vi "Button Toggle Motor.vi"(8 "error in (no error)":errorcluster, 9 "Motor Power":dbl format="%#_13g", 10 "refnum name":string="My Motor RefNum", 11 "Input":bool) -> (0 "error out":errorcluster)   [LabVIEW 2016, in "Huskie Swerve.lvlib"]
uses:
  Huskie Swerve.lvlib
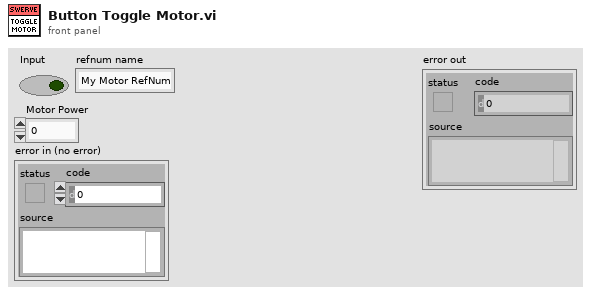
[diagram p1: front panel]
types:
  T1 = typedef "WPI_MotorControlDeviceRef.ctl" = cluster{"DeviceStatus":errorcluster, "Type":T2, "PWM":cluster{"PWM Channel":T3, "DeadBand":T4}, "CAN":cluster{"Device Number":u8, "SetOutput VI Ref":variant, "GetOutput VI Ref":variant, "Enable VI Ref":variant, "Disable VI Ref":variant, "Data":variant}, "Invert":bool}
  T2 = typedef "WPI_MotorControlType.ctl" = enum16{"PWM", "CAN"}
  T3 = typedef "FPGA_DIOPWMChannel.ctl" = enum8{"PWM 0", "PWM 1", "PWM 2", "PWM 3", "PWM 4", "PWM 5", "PWM 6", "PWM 7", "PWM 8", "PWM 9", "PWM MXP 0", "PWM MXP 1", "PWM MXP 2", "PWM MXP 3", "PWM MXP 4", "PWM MXP 5", "PWM MXP 6", "PWM MXP 7", "PWM MXP 8", "PWM MXP 9", "Invalid"}
  T4 = typedef "WPI_PWMDeadband.ctl" = cluster{"Name":string, "maxPositivePwm":i32, "minPositivePwm":i32, "centerPwm":i32, "maxNegativePwm":i32, "minNegativePwm":i32, "angularRange":u16}
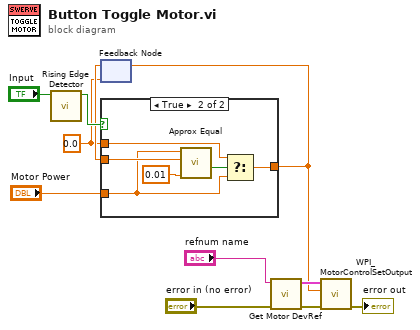
[diagram p0: block diagram]
diagram:
  w2 = 0.0 ("f")
  n1 = call "Rising Edge Detector.vi"("Input"="Input") -> ("Rising edge?"=w5:bool)  [unwired: 10 in]
  n2 = feedback #1(w2) -> (w4:dbl)
  n3 = case shown="True" w5 {
    tunnel: w4 -> [w12 w18]
    tunnel: "Motor Power" -> [_ w14]
    tunnel: w2 -> [_ w15]
    tunnel: [w12 w13] -> w1
    frame False {
    }
    frame True {
      n4 = call "Approx Equal.vi"("Tolerance"=0.01, "b"=w18, "a"=w14) -> ("a == b?"=w16:bool)  [unwired: 8 in]
      n5 = Select(t=w15, s=w16, f=w14) -> (s? t:f=w13:dbl)
    }
  }
  n6 = feedback-in #1(w1) -> ()
  n7 = call "Get Motor DevRef.vi"("error in (no error)"="error in (no error)", "refnum name"="refnum name") -> ("error out"=w8:errorcluster, "MotorControlDevRef"=w10:T1)  [unwired: 8 in]
  n8 = call <vilib>:"WPI_MotorControlSetOutput.vi"("error in (no error)"=w8, "Output"=w1, "MotorControlDevRef"=w10) -> ("error out"=→"error out":errorcluster)  [unwired: 6 in, 2 out]
